vi "SBML_Init_Assign.vi"(8 "error in (no error)":errorcluster, 11 "Input SBML File":string) -> (0 "error out":errorcluster, 2 "Initial Assignments":string[][](table), 3 "InitAssignCnt":i32)   [LabVIEW 2014]
doc: "This VI extract the information of species present in SBML file. It takes the complete SBML file as input, and outputs: \nSp_Cnt --> How many species are there\nS_Id_Arr --> Array of species\nSp_Name --> Array containing the name of species\nSp_Init_Amnt --> Array containing the initial amount of species\n\nDesigned by HB\nhaba@dtu.dk"
panel:
  out "Math":string[](array[string])
  out "Symbol":string[](array[string])
  out "List of Init Assign":string
  # "Names"
  # "Initial Amount"
  # "ID"
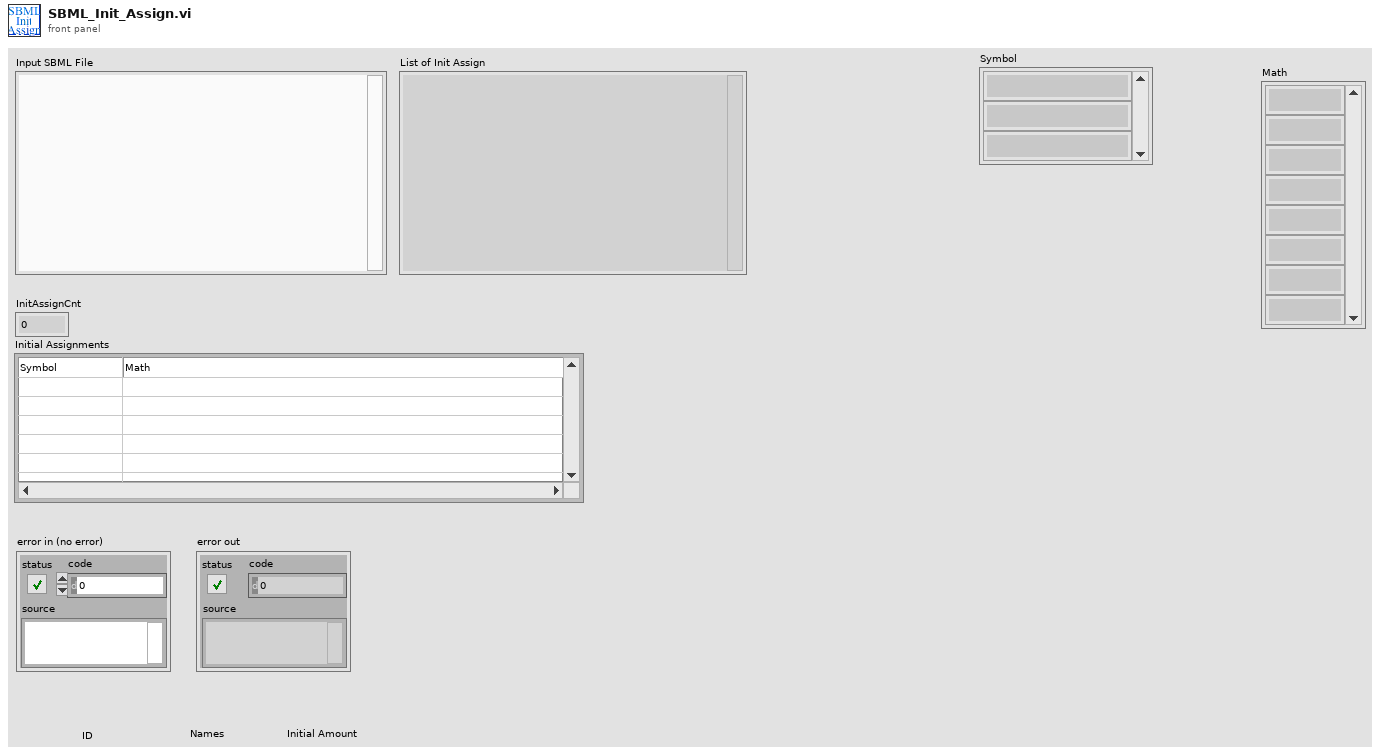
[diagram p1: front panel]
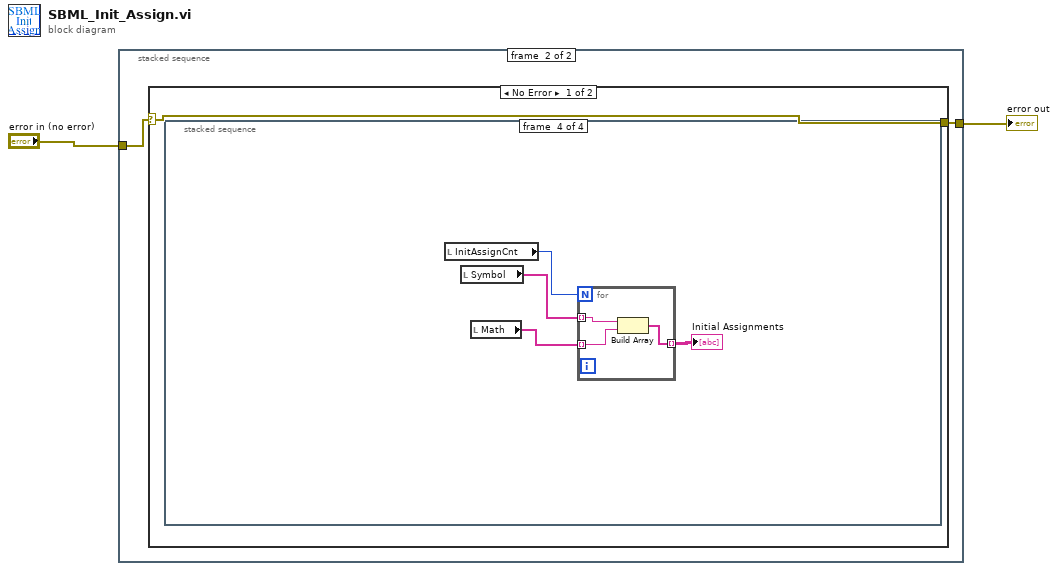
[diagram p0: block diagram]
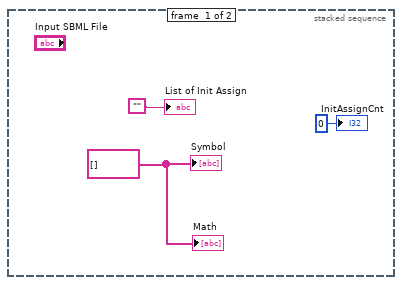
[diagram p2: hidden frame]
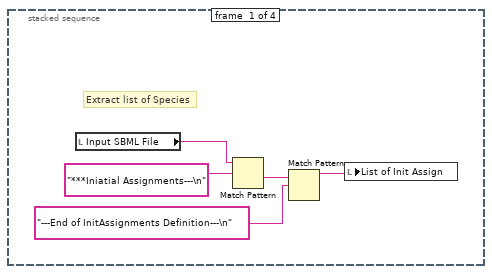
[diagram p3: hidden frame]
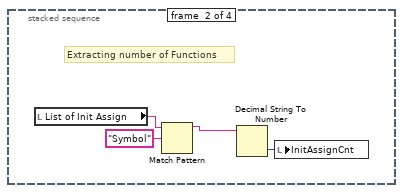
[diagram p4: hidden frame]
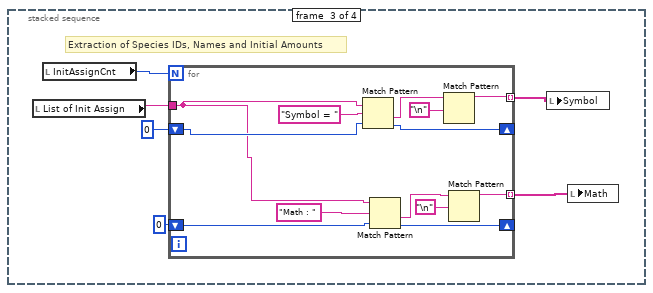
[diagram p5: hidden frame]
diagram:
  n1 = stacked-sequence {
    tunnel: "error in (no error)" -> [_ w6]
    tunnel: [_ w7] -> w1
    frame #0 {
      w3 = string[] [] ("Sp_Id_Arr")
      "List of Init Assign" <- "" ("Full SBML File")
      "InitAssignCnt" <- 0 ("Sp_cnt")
      "Symbol" <- w3
      "Math" <- w3
    }
    frame #1 {
      n2 = case shown="No Error" w6 {
        selector: w6 -> [w8 w44]
        tunnel: [w8 w44] -> w7
        frame No Error {
          n3 = stacked-sequence {
            frame #0 {
              # "Extract list of Species"
              n4 = local read "Input SBML File"() -> (w10:string)
              n5 = Match Pattern(string=w10, regular expression="***Iniatial Assignments---\n") -> (after substring=w12:string)  [unwired: 1 in, 3 out]
              n6 = Match Pattern(string=w12, regular expression="---End of InitAssignments Definition---\n") -> (before substring=w9:string)  [unwired: 1 in, 3 out]
              n7 = local write "List of Init Assign"(w9) -> ()
            }
            frame #1 {
              # "Extracting number of Functions"
              n8 = local read "List of Init Assign"() -> (w14:string)
              n9 = Match Pattern(string=w14, regular expression="Symbol") -> (before substring=w15:string)  [unwired: 1 in, 3 out]
              n10 = Decimal String To Number(string=w15) -> (number=w17:i32)  [unwired: 2 in, 1 out]
              n11 = local write "InitAssignCnt"(w17) -> ()
            }
            frame #2 {
              # "Extraction of Species IDs, Names and Initial Amounts"
              n12 = local read "List of Init Assign"() -> (w22:string)
              n13 = local read "InitAssignCnt"() -> (w21:i32)
              n14 = for {
                N: w21 -> [_]
                tunnel: w22 -> [w24]
                shift-right: [w31] -> _
                shift-left: 0 ("offset past match") -> [w32]
                tunnel: [w33] -> w20 mode=indexing
                shift-right: [w27] -> _
                shift-left: 0 ("offset past match") -> [w26]
                tunnel: [w25] -> w18 mode=indexing
                n15 = Match Pattern(string=w24, regular expression="Symbol = ", offset (0)=w32) -> (after substring=w34:string, offset past match=w31:i32)  [unwired: 2 out]
                n16 = Match Pattern(string=w24, regular expression="Math : ", offset (0)=w26) -> (after substring=w30:string, offset past match=w27:i32)  [unwired: 2 out]
                n17 = Match Pattern(string=w34, regular expression="\n") -> (before substring=w33:string)  [unwired: 1 in, 3 out]
                n18 = Match Pattern(string=w30, regular expression="\n") -> (before substring=w25:string)  [unwired: 1 in, 3 out]
              }
              n19 = local write "Symbol"(w20) -> ()
              n20 = local write "Math"(w18) -> ()
            }
            frame #3 {
              n21 = local read "InitAssignCnt"() -> (w38:i32)
              n22 = local read "Symbol"() -> (w37:string[])
              n23 = local read "Math"() -> (w39:string[])
              n24 = for {
                N: w38 -> [_]
                tunnel: w37 -> [w43] mode=indexing
                tunnel: [w42] -> w40 mode=indexing
                tunnel: w39 -> [w41] mode=indexing
                n25 = Build Array(w43, w41) -> (w42:string[])
              }
              "Initial Assignments" <- w40
            }
          }
        }
        frame Error {
        }
      }
    }
  }
  "error out" <- w1
